vi "写入命令.vi"(8 "error in (no error)":errorcluster caption="错误输入（无错误）", 10 "字符串":string, 11 "A命令 输入":refnum<class "A命令.lvclass">) -> (0 "error out":errorcluster caption="错误输出", 3 "A命令 输出":refnum<class "A命令.lvclass">)   [LabVIEW 2016, in "A命令.lvclass"]
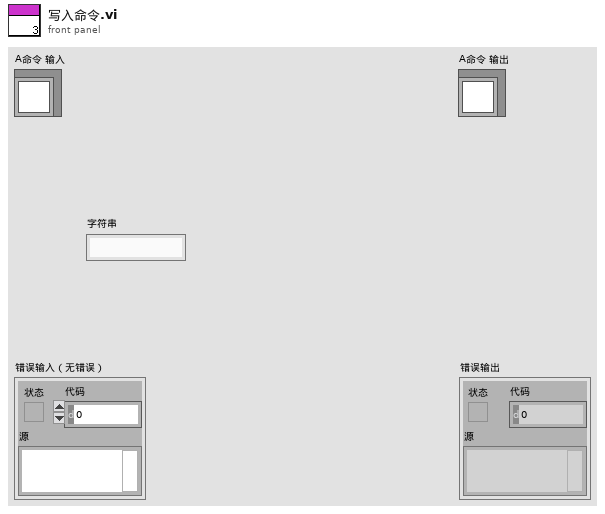
[diagram p1: front panel]
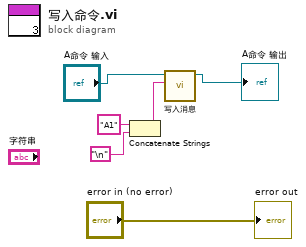
[diagram p0: block diagram]
diagram:
  n1 = Concatenate Strings("A1" ("字符串"), "\n") -> (w2:string)
  n2 = call-dynamic "写入消息.vi"("消息"=w2, "消息类输入"="A命令 输入") -> ("消息类输出"=→"A命令 输出":refnum<class "A命令.lvclass">)  [unwired: 8 in, 1 out]
  "error out" <- "error in (no error)"
